vi "MIMIC Commands Rev 6.vi"(6 "MIMIC HOST COMMAND":T2(ring)=enum."Read Serial Number", 8 "Input String Data Array":string[](array[string])=["1"], 9 "HWHSflag":bool, 10 "wait (ms)":u32=500, 11 "VISA resource name":refnum<visa-resource-name>="COM5") -> (0 "error out":errorcluster={"status"=FALSE, "code"=1073676294, "source"="VISA Read in MIMIC RecvCommand.vi->MIMIC Commands Rev 2.vi"}, 1 "Receive_buffer":u8[](array[numeric]) format="%x", 2 "Receive_Unpacked_Data":T1)   [LabVIEW 2014]
panel:
  out "local":i32
  out "GUID":string
  out "Array":u8[](array[numeric]) format="%x"
  out "TimeToDecode":u16
  out "VISA resource name OUT":refnum<visa-resource-name>="COM5"
  out "hex integer string":string[](array[string])=["4", "D0", "0", "0", "FF", "2C"]
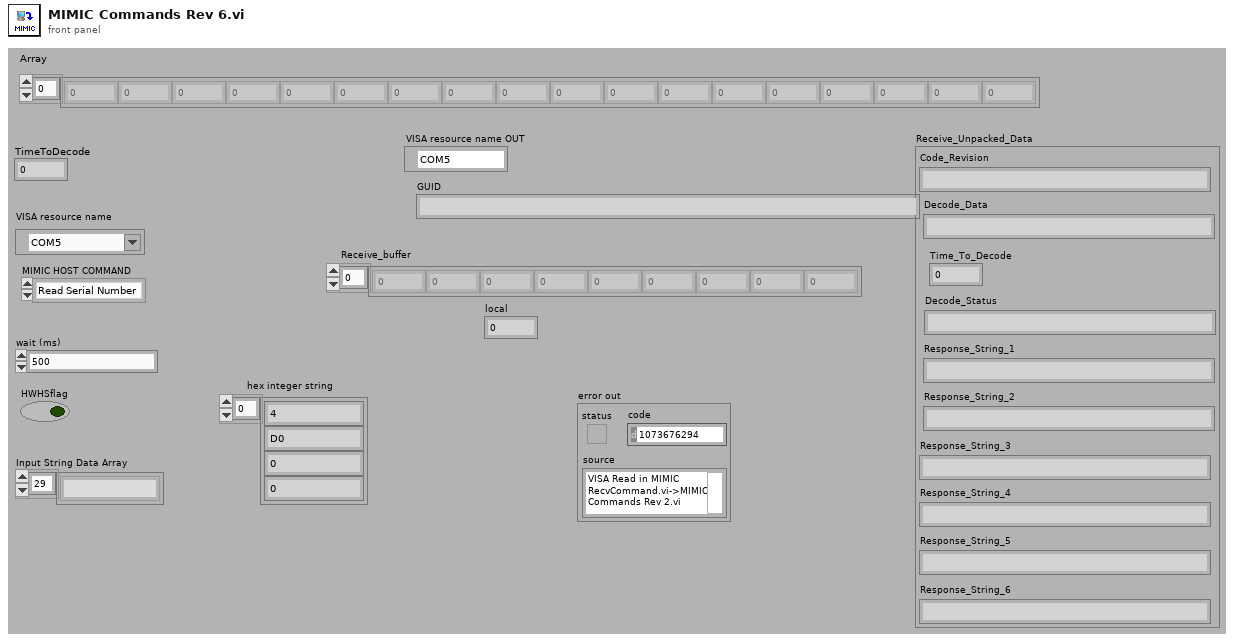
[diagram p1: front panel]
types:
  T1 = cluster{"Code_Revision":string, "Decode_Data":string, "Decode_Status":string, "Response_String_1":string, "Response_String_2":string, "Response_String_3":string, "Response_String_4":string, "Response_String_5":string, "Response_String_6":string, "Time_To_Decode":u16}
  T2 = enum16{"Enter FAT", "Beeper Control", "LED Off", "LED On", "Image Mode", "Start Session", "Stop Session", "Change Buadrate", "Auto Exposure", "Set Manual Exposure", "Read BT Address", "Store BT Address", "Pairing Command", "Query Paired Address", "Pairing Status", "Un-Pairing", "Set Illumination", "Trigger", "Set Defaults", "Imager Time To Decode Test", "Battery Off", "Battery Charge Control", "Read Battery Voltage", "Read Battery Temperature", "Software Version", "StoreFeatureSet", "ReadFeatureSet", "Store Model Number", "Read Model Number", "Store Manufacturing Date", "Read Manufacturing Date", "Store Service Date", "Read Service Date", "Store Serial Number", "Read Serial Number", "Exit FAT", "Read GUID", "Cable Auto ID", "Store RSM 627", "Read RSM 627", "Hall Effect switch", "Store GUID ", "ParamSend", "General", "General-Response", "RSM Init", "RSM EnterFAT", "RSM - SE4500 - Peek PRISM Register GENERIC command", "RSM - SE4500 - Poke PRISM Register GENERIC command", "RSM - SE4500 - GENERIC command", "RSM - SE4500 - GetPDM Calibration", "RSM - SE4500 - SetPDM Calibration", "Get Object Sensor Value", "Store Object Sensor Calibration Value", "Read Object Sensor Calibration Value", "RSM - SE4500 - GetPDM-Z Calibration", "RSM - SE4500 - SetPDM-Z Calibration", "Store FIPSKEY", "Read FIPSKEY"}
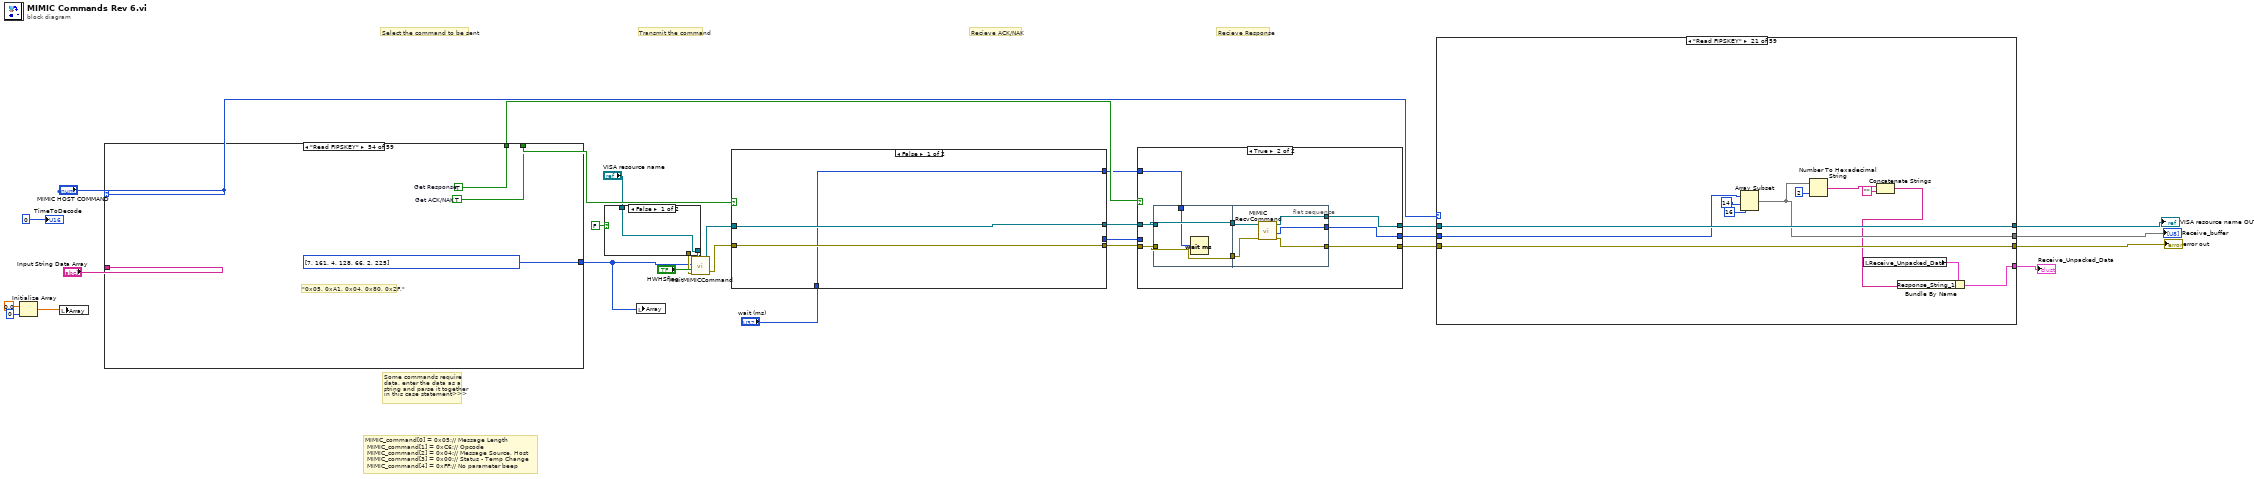
[diagram p0: block diagram]
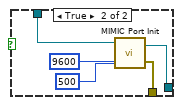
[diagram p2: hidden frame]
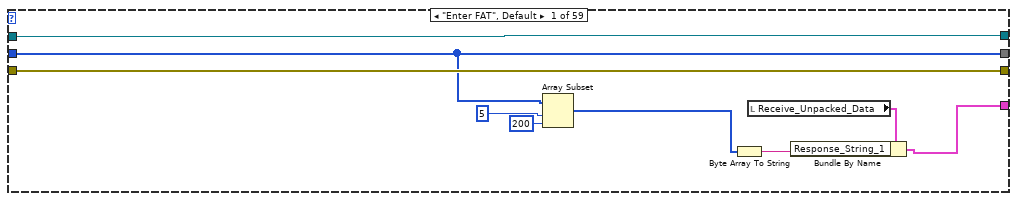
[diagram p3: hidden frame]
diagram:
  # "MIMIC_command[0] = 0x05;// Message Length \n\tMIMIC_command[1] = 0xC6;// Opcode  \n\tMIMIC_command[2] = 0x04;// Message Source, Host \n\tMIMIC_command[3] = 0x00;// Status - Temp Change            \n\tMIMIC_command[4] = 0xFF;// No parameter beep"
  # "Transmit the command"
  # "Recieve Response"
  # "Recieve ACK/NAK"
  # "Select the command to be sent"
  # "Some commands require\ndata, enter the data as a\nstring and parse it together\nin this case statement>>>"
  n1 = Initialize Array(0.0 ("element"), 0 ("dimension size")) -> (w5:dbl[])
  n2 = local write "Array"(w5) -> ()
  n3 = case shown="\"Read FIPSKEY\"" "MIMIC HOST COMMAND" {
    tunnel: "Input String Data Array" -> [w37 w39 w62 _ _ _ _ _ w86 w113 w139 w179 w219 w256 _ _ _ w274 w290 w300 w315 w328 w346 w362 _ _ _ _ _ w386 _ _ _ w406 _ _ _ _ w431 _ w443 _ w453 _ _ _ w479 _ w491 _ _ _ _ _ _ _ _ _ _]
    tunnel: [w31 w45 w66 u8[] [5, 161, 4, 128, 16, 0, 0, 0, 0, 0, 0, 0, 0, 0] u8[] [14, 128, 4, 0, 0, 10, 112, 0, 1, 20, 112, 12, 0, 132] u8[] [14, 128, 4, 0, 0, 10, 112, 0, 1, 20, 112, 31, 0, 113] u8[] [12, 128, 4, 0, 0, 6, 32, 0, 0, 240, 0, 0, 0, 0] u8[] [13, 128, 4, 0, 0, 9, 112, 0, 1, 2, 120, 1, 135, 0] w85 w119 w140 w176 w217 w257 u8[] [4, 228, 4, 0, 0, 0, 0, 0, 0, 0, 0, 0, 0, 0] u8[] [4, 228, 4, 0, 0, 0, 0, 0, 0, 0, 0, 0, 0, 0] u8[] [7, 215, 4, 0, 4, 11, 0, 255, 15, 0, 0, 0, 0, 0] w275 w284 w298 w313 w332 w349 w361 u8[] [16, 161, 4, 128, 16, 0, 0, 0, 0, 0, 0, 0, 0, 0] u8[] [5, 161, 4, 128, 16, 0, 0, 0, 0, 0, 0, 0, 0, 0] u8[] [4, 200, 4, 128, 0, 0, 0, 0, 0, 0, 0, 0, 0, 0] u8[] [5, 161, 4, 128, 25, 0, 0, 0, 0, 0, 0, 0, 0, 0] u8[] [7, 161, 4, 128, 66, 2, 29, 0, 0, 0, 0, 0, 0, 0] w385 u8[] [6, 161, 4, 128, 45, 2, 0, 0, 0, 0, 0, 0, 0, 0] u8[] [7, 161, 4, 128, 48, 19, 136, 0, 0, 0, 0, 0, 0, 0] u8[] [5, 161, 4, 128, 60, 0, 0, 0, 0, 0, 0, 0, 0, 0] w405 u8[] [7, 161, 4, 128, 66, 117, 48, 0, 0, 0, 0, 0, 0, 0] u8[] [7, 161, 4, 128, 66, 117, 49, 0, 0, 0, 0, 0, 0, 0] u8[] [7, 161, 4, 128, 66, 78, 41, 0, 0, 0, 0, 0, 0, 0] u8[] [6, 161, 4, 128, 96, 8] w424 u8[] [7, 161, 4, 128, 66, 3, 36] w445 u8[] [7, 161, 4, 128, 66, 2, 194, 0, 0, 0, 0, 0, 0, 0] w458 u8[] [7, 161, 4, 128, 66, 2, 21, 0, 0, 0, 0, 0, 0, 0] w472 u8[] [7, 161, 4, 128, 66, 2, 23, 0, 0, 0, 0, 0, 0, 0] w484 u8[] [7, 161, 4, 128, 66, 2, 24, 0, 0, 0, 0, 0, 0, 0] w496 u8[] [7, 161, 4, 128, 66, 2, 22, 0, 0, 0, 0, 0, 0, 0] u8[] [5, 161, 4, 128, 54, 254, 160, 0, 0, 0, 0, 0, 0, 0] u8[] [5, 161, 4, 128, 84, 0, 0, 0, 0, 0, 0, 0, 0, 0] u8[] [5, 161, 4, 128, 47] u8[] [7, 161, 4, 128, 66, 2, 225] w514 u8[] [5, 161, 4, 128, 110] u8[] [10, 161, 4, 128, 69, 2, 115, 66, 7, 2] u8[] [6, 161, 4, 128, 45, 1, 0, 0, 0, 0, 0, 0, 0, 0] u8[] [7, 161, 4, 128, 66, 2, 115]] -> w6
    tunnel: [w30 w57 w64 w71 w75 w78 w81 w84 w108 w135 w172 w192 w232 w258 w266 w269 w271 w276 w291 w301 w316 w333 w350 w368 w371 w373 w376 w380 w384 w388 w395 w399 w402 w403 w414 w417 w419 w422 w437 w440 w448 w451 w457 w462 w471 w476 w483 w487 w494 w499 w503 w507 w508 w511 w519 w521 w524 w527 w531] -> w25
    tunnel: [w29 w56 w65 w70 w74 w77 w80 w83 w107 w134 w171 w191 w231 w259 w267 w270 w272 w277 w292 w302 w317 w334 w351 w369 w372 w374 w377 w379 w383 w387 w396 w398 w401 w404 w413 w416 w418 w421 w436 w439 w447 w450 w456 w463 w470 w475 w482 w488 w495 w500 w502 w506 w509 w512 w520 w522 w525 w528 w530] -> w27
    frame "LED On" {
      w30 = FALSE  # Get Response
      w29 = TRUE  # Get ACK/NAK
      # "LED data Byte"
      n4 = Index Array(array=w37, index=0) -> (element=w36:string)
      n5 = Decimal String To Number(string=w36) -> (number=w35:i32)  [unwired: 2 in, 1 out]
      n6 = Replace Array Subset(array=u8[] [5, 231, 4, 128, 1, 0, 0, 0, 0, 0, 0, 0, 0, 0], new element=w35, index=4) -> (w31:u8[])
    }
    frame "ParamSend" {
      w57 = FALSE  # Get Response
      w56 = TRUE  # Get ACK/NAK
      n7 = Array Size(array=w39) -> (size(s)=w38:i32)
      n8 = Index Array(array=w39, index=0) -> (element=w61:string)
      n9 = Add(x=w38, y=5) -> (x+y=w43:i32)
      n10 = Hexadecimal String To Number(string=w61) -> (number=w42:u32)  [unwired: 2 in, 1 out]
      n11 = Replace Array Subset(array=u8[] [5, 198, 4, 128, 255, 0, 0, 0, 0, 0, 0, 0, 0, 0], new element=w43, index=0) -> (w54:u8[])
      n12 = Replace Array Subset(array=w54, new element=w42, index=5) -> (w50:u8[])
      n13 = Index Array(array=w39, index=2) -> (element=w49:string)
      n14 = Index Array(array=w39, index=1) -> (element=w53:string)
      n15 = Hexadecimal String To Number(string=w49) -> (number=w40:u32)  [unwired: 2 in, 1 out]
      n16 = Hexadecimal String To Number(string=w53) -> (number=w41:u32)  [unwired: 2 in, 1 out]
      n17 = Replace Array Subset(array=w50, new element=w41, index=6) -> (w46:u8[])
      n18 = Replace Array Subset(array=w46, new element=w40, index=7) -> (w45:u8[])
    }
    frame "Beeper Control" {
      w64 = FALSE  # Get Response
      w65 = TRUE  # Get ACK/NAK
      # "Beeper data Byte"
      n19 = Decimal String To Number(string=w62, offset=0) -> (number=w69:i32[])  [unwired: 1 in, 1 out]
      n20 = Replace Array Subset(array=u8[] [5, 230, 4, 128, 0, 0, 0, 0, 0, 0, 0, 0, 0, 0], new element=w69, index=4) -> (w66:u8[])
    }
    frame "Enter FAT" {
      w71 = TRUE  # Get Response
      w70 = TRUE  # Get ACK/NAK
      # "Enter FAT command:\n0x05:0xA1:0x40:0x80:0x10"
    }
    frame "RSM - SE4500 - GetPDM Calibration" {
      w75 = TRUE  # Get Response
      w74 = FALSE  # Get ACK/NAK
      # "RSM GetDPMCalibration Command"
    }
    frame "RSM - SE4500 - GetPDM-Z Calibration" {
      w78 = TRUE  # Get Response
      w77 = FALSE  # Get ACK/NAK
      # "RSM GetDPMCalibration Command"
    }
    frame "RSM Init" {
      w81 = TRUE  # Get Response
      w80 = FALSE  # Get ACK/NAK
      # "Init RSM command:\n0x0C:0x80:0x04:0x00:0x00:0x06:0x20:0x00:0x00:0xF0"
    }
    frame "RSM EnterFAT" {
      w84 = TRUE  # Get Response
      w83 = FALSE  # Get ACK/NAK
      # "RSM / SE4500 - Enter FAT command:\n0x0D:0x80:0x04:0x00:0x00:0x09:0x70:0x00:0x01:0x02:0x78:0x01:0x87:"
    }
    frame "RSM - SE4500 - Peek PRISM Register GENERIC command" {
      w108 = TRUE  # Get Response
      w107 = FALSE  # Get ACK/NAK
      # "Register Word - HEX String"
      # "RSM / SE4500 - Peek PRISM Register GENERIC command:\n0x0E:0x80:0x04:0x00:0x00:0x0B:0x70:0x00:0x01:0x02:0xC3:0xXX:0xXX:0xXX:0xCS"
      n21 = Index Array(array=w86, index=0) -> (element=w90:string)
      n22 = Hexadecimal String To Number(string=w90, default (0uL)=i16 0 ("default (0 I32)")) -> (number=w88:i16)  [unwired: 1 in, 1 out]
      n23 = Split Number(x=w88) -> (hi(x)=w94:u8, lo(x)=w92:u8)
      n24 = Replace Array Subset(array=u8[] [15, 128, 4, 0, 0, 11, 112, 0, 1, 3, 195, 0, 0, 0, 0], new element=w94, index=11) -> (w91:u8[])
      n25 = Replace Array Subset(array=w91, new element=w92, index=12) -> (w87:u8[])
      n26 = Array Subset(array=w87, index=10, length=3) -> (w97:u8[])
      n27 = for {
        N: 3 -> [_]
        tunnel: w97 -> [w111] mode=indexing
        shift-right: [w109] -> w103
        shift-left: u16 0 -> [w110]
        n28 = Add(x=w110, y=w111) -> (x+y=w109:u16)
      }
      n29 = Not(x=w103) -> (.not. x?=w102:u16)
      n30 = Increment(x=w102) -> (x+1=w101:u16)
      n31 = Replace Array Subset(array=w87, new element=w101, index=13) -> (w85:u8[])
    }
    frame "RSM - SE4500 - GENERIC command" {
      w114 = 1 ("index")
      w118 = 0 ("index")
      w135 = TRUE  # Get Response
      w134 = FALSE  # Get ACK/NAK
      # "Register Word - HEX String"
      # "RSM / SE4500 - Peek PRISM Register GENERIC command:\n0x0E:0x80:0x04:0x00:0x00:0x0B:0x70:0x00:0x01:0x02:0xXX:0xXX:0xXX:0xCS"
      n32 = Index Array(array=w113, index=w118) -> (element=w121:string)
      n33 = Index Array(array=w113, index=w114) -> (element=w115:string)
      n34 = Hexadecimal String To Number(string=w121, default (0uL)=w118) -> (number=w116:i32)  [unwired: 1 in, 1 out]
      n35 = Hexadecimal String To Number(string=w115, default (0uL)=w114) -> (number=w112:i32)  [unwired: 1 in, 1 out]
      n36 = Replace Array Subset(array=u8[] [13, 128, 4, 0, 0, 9, 112, 0, 1, 2, 255, 0, 0], new element=w116, index=10) -> (w122:u8[])
      n37 = Replace Array Subset(array=w122, new element=w112, index=11) -> (w120:u8[])
      n38 = Array Subset(array=w120, index=10, length=2) -> (w125:u8[])
      n39 = for {
        N: 2 -> [_]
        tunnel: w125 -> [w138] mode=indexing
        shift-right: [w136] -> w131
        shift-left: u16 0 -> [w137]
        n40 = Add(x=w137, y=w138) -> (x+y=w136:u16)
      }
      n41 = Not(x=w131) -> (.not. x?=w130:u16)
      n42 = Increment(x=w130) -> (x+1=w129:u16)
      n43 = Replace Array Subset(array=w120, new element=w129, index=12) -> (w119:u8[])
    }
    frame "RSM - SE4500 - Poke PRISM Register GENERIC command" {
      w172 = TRUE  # Get Response
      w171 = FALSE  # Get ACK/NAK
      # "Register Word - HEX String"
      # "Register Word - HEX String"
      # "Value Byte - Decimal String"
      # "RSM / SE4500 - Poke PRISM Register GENERIC command:\n0x0E:0x80:0x04:0x00:0x00:0x0B:0x70:0x00:0x01:0x02:0xC0:0xXX:0xXX:0xXX:0xCS"
      n44 = Index Array(array=w139, index=0) -> (element=w154:string)
      n45 = Index Array(array=w139, index=1) -> (element=w145:string)
      n46 = Hexadecimal String To Number(string=w154, default (0uL)=i16 0 ("default (0 I32)")) -> (number=w152:i16)  [unwired: 1 in, 1 out]
      n47 = Split Number(x=w152) -> (hi(x)=w158:u8, lo(x)=w156:u8)
      n48 = Hexadecimal String To Number(string=w145, default (0uL)=i16 0 ("default (0 I32)")) -> (number=w151:i16)  [unwired: 1 in, 1 out]
      n49 = Replace Array Subset(array=u8[] [16, 128, 4, 0, 0, 12, 112, 0, 1, 2, 151, 0, 0, 0, 0, 0], new element=w158, index=12) -> (w155:u8[])
      n50 = Split Number(x=w151) -> (hi(x)=w148:u8, lo(x)=w150:u8)
      n51 = Replace Array Subset(array=w155, new element=w156, index=11) -> (w143:u8[])
      n52 = Replace Array Subset(array=w143, new element=w148, index=14) -> (w142:u8[])
      n53 = Replace Array Subset(array=w142, new element=w150, index=13) -> (w141:u8[])
      n54 = Array Subset(array=w141, index=10, length=5) -> (w161:u8[])
      n55 = for {
        N: 5 -> [_]
        tunnel: w161 -> [w175] mode=indexing
        shift-right: [w173] -> w167
        shift-left: u16 0 -> [w174]
        n56 = Add(x=w174, y=w175) -> (x+y=w173:u16)
      }
      n57 = Not(x=w167) -> (.not. x?=w166:u16)
      n58 = Increment(x=w166) -> (x+1=w165:u16)
      n59 = Replace Array Subset(array=w141, new element=w165, index=15) -> (w140:u8[])
    }
    frame "RSM - SE4500 - SetPDM Calibration" {
      w192 = TRUE  # Get Response
      w191 = FALSE  # Get ACK/NAK
      # "RSM / SE4500 - SetDPMCalibration command:"
      n60 = for {
        N: 8 -> [_]
        shift-right: [w202] -> w178
        shift-left: u8[] [30, 128, 4, 0, 0, 26, 112, 0, 1, 2, 148, 12, 0, 0, 0, 0, 0, 0, 0, 0, 0, 0, 0, 0, 0, 0, 0, 0, 0, 0, 0] -> [w209]
        tunnel: w179 -> [w208]
        i -> [w204]
        # "high byte"
        # "low byte"
        n61 = Index Array(array=w208, index=w204) -> (element=w197:string)
        n62 = Decimal String To Number(string=w197, default (0L)=0 ("default (0 I32)")) -> (number=w194:i32)  [unwired: 1 in, 1 out]
        n63 = Number To Hexadecimal String(1:i16 4 ("width (-)"), 2:w194) -> (0:w195:string)
        n64 = local read "local"() -> (w200:i32)
        n65 = Hexadecimal String To Number(string=w195, default (0uL)=i16 0 ("default (0 I32)")) -> (number=w210:i16)  [unwired: 1 in, 1 out]
        n66 = Add(x=1 ("y"), y=w200) -> (x+y=w198:i32)
        n67 = Add(x=w204, y=w198) -> (x+y=w201:i32)
        n68 = Add(x=1 ("index"), y=w201) -> (x+y=w206:i32)
        n69 = Split Number(x=w210) -> (hi(x)=w212:u8, lo(x)=w211:u8)
        n70 = Replace Array Subset(array=w209, new element=w212, index=w206) -> (w203:u8[])
        n71 = local write "local"(w198) -> ()
        n72 = Replace Array Subset(array=w203, new element=w211, index=w201) -> (w202:u8[])
      }
      n73 = Array Subset(array=w178, index=10, length=19) -> (w182:u8[])
      n74 = for {
        N: 19 -> [_]
        tunnel: w182 -> [w215] mode=indexing
        shift-right: [w213] -> w188
        shift-left: u16 0 -> [w214]
        n75 = Add(x=w214, y=w215) -> (x+y=w213:u16)
      }
      n76 = Not(x=w188) -> (.not. x?=w187:u16)
      n77 = Increment(x=w187) -> (x+1=w186:u16)
      n78 = Replace Array Subset(array=w178, new element=w186, index=29) -> (w176:u8[])
      "local" <- 12 ("x+y")
    }
    frame "RSM - SE4500 - SetPDM-Z Calibration" {
      w232 = TRUE  # Get Response
      w231 = FALSE  # Get ACK/NAK
      # "RSM / SE4500 - SetDPMCalibration command:"
      n79 = local write "local"(12 ("x+y")) -> ()
      n80 = for {
        N: 8 -> [_]
        shift-right: [w242] -> w218
        shift-left: u8[] [30, 128, 4, 0, 0, 26, 112, 0, 1, 2, 148, 31, 0, 0, 0, 0, 0, 0, 0, 0, 0, 0, 0, 0, 0, 0, 0, 0, 0, 0, 0] -> [w249]
        tunnel: w219 -> [w248]
        i -> [w244]
        # "high byte"
        # "low byte"
        n81 = Index Array(array=w248, index=w244) -> (element=w237:string)
        n82 = Decimal String To Number(string=w237, default (0L)=0 ("default (0 I32)")) -> (number=w234:i32)  [unwired: 1 in, 1 out]
        n83 = Number To Hexadecimal String(1:i16 4 ("width (-)"), 2:w234) -> (0:w235:string)
        n84 = local read "local"() -> (w240:i32)
        n85 = Hexadecimal String To Number(string=w235, default (0uL)=i16 0 ("default (0 I32)")) -> (number=w250:i16)  [unwired: 1 in, 1 out]
        n86 = Add(x=1 ("y"), y=w240) -> (x+y=w238:i32)
        n87 = Add(x=w244, y=w238) -> (x+y=w241:i32)
        n88 = Add(x=1 ("index"), y=w241) -> (x+y=w246:i32)
        n89 = Split Number(x=w250) -> (hi(x)=w252:u8, lo(x)=w251:u8)
        n90 = Replace Array Subset(array=w249, new element=w252, index=w246) -> (w243:u8[])
        n91 = local write "local"(w238) -> ()
        n92 = Replace Array Subset(array=w243, new element=w251, index=w241) -> (w242:u8[])
      }
      n93 = Array Subset(array=w218, index=10, length=19) -> (w222:u8[])
      n94 = for {
        N: 19 -> [_]
        tunnel: w222 -> [w255] mode=indexing
        shift-right: [w253] -> w228
        shift-left: u16 0 -> [w254]
        n95 = Add(x=w254, y=w255) -> (x+y=w253:u16)
      }
      n96 = Not(x=w228) -> (.not. x?=w227:u16)
      n97 = Increment(x=w227) -> (x+1=w226:u16)
      n98 = Replace Array Subset(array=w218, new element=w226, index=29) -> (w217:u8[])
    }
    frame "Image Mode" {
      w258 = FALSE  # Get Response
      w259 = TRUE  # Get ACK/NAK
      # "Image Mode Byte:\n00: Decode\n01: SnapShot\n02: Video\n03: Last Decode\n04: las No Decode"
      n99 = Index Array(array=w256, index=0) -> (element=w264:string)
      n100 = Decimal String To Number(string=w264) -> (number=w263:i32)  [unwired: 2 in, 1 out]
      n101 = Replace Array Subset(array=u8[] [5, 247, 4, 128, 0, 0, 0, 0, 0, 0, 0, 0, 0, 0], new element=w263, index=4) -> (w257:u8[])
    }
    frame "Start Session" {
      w266 = FALSE  # Get Response
      w267 = TRUE  # Get ACK/NAK
      # "Start Session"
    }
    frame "Stop Session" {
      w269 = FALSE  # Get Response
      w270 = TRUE  # Get ACK/NAK
      # "Start Session"
    }
    frame "Change Buadrate" {
      w271 = FALSE  # Get Response
      w272 = FALSE  # Get ACK/NAK
      # "Enter FAT command:\n06: 9600\n08: 38400\n0A: 57600\n0B:115200\n0C:230400"
    }
    frame "Auto Exposure" {
      w276 = FALSE  # Get Response
      w277 = TRUE  # Get ACK/NAK
      # "Auto Exposure:\n00:Disabled\n01: Enabled"
      n102 = Index Array(array=w274, index=0) -> (element=w282:string)
      n103 = Decimal String To Number(string=w282) -> (number=w281:i32)  [unwired: 2 in, 1 out]
      n104 = Replace Array Subset(array=u8[] [8, 198, 4, 0, 255, 240, 41, 0, 0, 0, 0, 0, 0, 0], new element=w281, index=7) -> (w275:u8[])
    }
    frame "Set Manual Exposure" {
      w291 = FALSE  # Get Response
      w292 = TRUE  # Get ACK/NAK
      # "Image Mode Byte:\n00: Decode\n01: SnapShot\n02: Video\n03: Last Decode\n04: las No Decode"
      n105 = Index Array(array=w290, index=0) -> (element=w296:string)
      n106 = Decimal String To Number(string=w296, default (0L)=u16 0 ("default (0 I32)")) -> (number=w289:u16)  [unwired: 1 in, 1 out]
      n107 = Split Number(x=w289) -> (hi(x)=w287:u8, lo(x)=w286:u8)
      n108 = Replace Array Subset(array=u8[] [10, 198, 4, 0, 255, 244, 241, 55, 0, 0, 0, 0, 0, 0], new element=w287, index=8) -> (w283:u8[])
      n109 = Replace Array Subset(array=w283, new element=w286, index=9) -> (w284:u8[])
    }
    frame "Store BT Address" {
      w301 = FALSE  # Get Response
      w302 = TRUE  # Get ACK/NAK
      # "Store BT command:\n0x16, 0xA1, 0x04, 0x80, 0x45, 0x02, 0x1D, 0x41, 0x07, 0x42, 0x00, 0x06, 0x00, 0x00, \n\t\t\t\t\t\t\t\t\t\t0x00, 0x00, 0x00, 0x00, 0x00, 0x00,0x00, 0x00, 0xFF, 0xFF};"
      n110 = for {
        N: 6 -> [_]
        tunnel: w300 -> [w311]
        tunnel: [w306] -> w298
        i -> [w308]
        n111 = Index Array(array=w311, index=w308) -> (element=w305:string)
        n112 = Add(x=14 ("index"), y=w308) -> (x+y=w309:i32)
        n113 = Hexadecimal String To Number(string=w305, offset=0) -> (number=w303:u32)  [unwired: 1 in, 1 out]
        n114 = local read "Array"() -> (w307:u8[])
        n115 = Replace Array Subset(array=w307, new element=w303, index=w309) -> (w306:u8[])
        n116 = local write "Array"(w306) -> ()
      }
      "Array" <- u8[] [22, 161, 4, 128, 69, 2, 29, 65, 7, 66, 0, 6, 0, 0, 0, 0, 0, 0, 0, 0, 255, 255, 255, 0, 0, 0, 0, 0, 0, 0, 0, 0, 0, 0, 0, 0, 0, 0, 0, 0, 0, 0, 0, 0, 0, 0, 0, 0, 0, 0, 0]
    }
    frame "Store FIPSKEY" {
      w316 = FALSE  # Get Response
      w317 = TRUE  # Get ACK/NAK
      # "Store BT command:\n0x20, 0xA1, 0x04, 0x80, 0x45, 0x02, 0xE1, 0x41, 0x07, 0x42, 0x00, 0x16, 0x00, 0x00,"
      n117 = for {
        N: 16 -> [_]
        tunnel: w315 -> [w326]
        tunnel: [w321] -> w313
        i -> [w323]
        n118 = Index Array(array=w326, index=w323) -> (element=w320:string)
        n119 = Add(x=14 ("index"), y=w323) -> (x+y=w324:i32)
        n120 = Hexadecimal String To Number(string=w320, offset=0) -> (number=w318:u32)  [unwired: 1 in, 1 out]
        n121 = local read "Array"() -> (w322:u8[])
        n122 = Replace Array Subset(array=w322, new element=w318, index=w324) -> (w321:u8[])
        n123 = local write "Array"(w321) -> ()
      }
      n124 = local write "Array"(u8[] [32, 161, 4, 128, 69, 2, 225, 65, 7, 66, 0, 22, 0, 0, 0, 0, 0, 0, 0, 0, 255, 255, 255, 0, 0, 0, 0, 0, 0, 0, 0, 0, 0, 0, 0, 0, 0, 0, 0, 0, 0, 0, 0, 0, 0, 0, 0, 0, 0, 0, 0]) -> ()
    }
    frame "General" {
      w330 = 0 ("offset")
      w333 = FALSE  # Get Response
      w334 = TRUE  # Get ACK/NAK
      # "Gneral FAT command:\n0x16, 0xA1, 0x04, 0x80, 0x45, 0x02, 0x1D, 0x41, 0x07, 0x42, 0x00, 0x06, 0x00, 0x00, \n\t\t\t\t\t\t\t\t\t\t0x00, 0x00, 0x00, 0x00, 0x00, 0x00,0x00, 0x00, 0xFF, 0xFF};"
      n125 = Index Array(array=w328, index=w330) -> (element=w329:string)
      n126 = Hexadecimal String To Number(string=w329, offset=w330) -> (number=w327:u32)  [unwired: 1 in, 1 out]
      n127 = for {
        N: w327 -> [_]
        tunnel: w328 -> [w343]
        tunnel: [w338] -> w332
        i -> [w340]
        n128 = Index Array(array=w343, index=w340) -> (element=w337:string)
        n129 = Add(x=0 ("index"), y=w340) -> (x+y=w341:i32)
        n130 = Hexadecimal String To Number(string=w337, offset=0) -> (number=w335:u32)  [unwired: 1 in, 1 out]
        n131 = local read "Array"() -> (w339:u8[])
        n132 = Replace Array Subset(array=w339, new element=w335, index=w341) -> (w338:u8[])
        n133 = local write "Array"(w338) -> ()
      }
      n134 = local write "Array"(u8[] [22, 0, 0, 0, 0, 0, 0, 0, 0, 0, 0, 0, 0, 0, 0, 0, 0, 0, 0, 0, 0, 0, 0, 0, 0, 0, 0, 0, 0, 0, 0, 0, 0, 0, 0, 0, 0, 0, 0, 0, 0, 0, 0, 0, 0, 0, 0, 0, 0, 0, 0]) -> ()
    }
    frame "General-Response" {
      w345 = 0 ("offset")
      w350 = TRUE  # Get Response
      w351 = TRUE  # Get ACK/NAK
      # "Gneral FAT command:\n0x16, 0xA1, 0x04, 0x80, 0x45, 0x02, 0x1D, 0x41, 0x07, 0x42, 0x00, 0x06, 0x00, 0x00, \n\t\t\t\t\t\t\t\t\t\t0x00, 0x00, 0x00, 0x00, 0x00, 0x00,0x00, 0x00, 0xFF, 0xFF};"
      n135 = Index Array(array=w346, index=w345) -> (element=w344:string)
      n136 = Hexadecimal String To Number(string=w344, offset=w345) -> (number=w347:u32)  [unwired: 1 in, 1 out]
      n137 = for {
        N: w347 -> [_]
        tunnel: w346 -> [w360]
        tunnel: [w355] -> w349
        i -> [w357]
        n138 = Index Array(array=w360, index=w357) -> (element=w354:string)
        n139 = Add(x=0 ("index"), y=w357) -> (x+y=w358:i32)
        n140 = Hexadecimal String To Number(string=w354, offset=0) -> (number=w352:u32)  [unwired: 1 in, 1 out]
        n141 = local read "Array"() -> (w356:u8[])
        n142 = Replace Array Subset(array=w356, new element=w352, index=w358) -> (w355:u8[])
        n143 = local write "Array"(w355) -> ()
      }
      n144 = local write "Array"(u8[] [22, 0, 0, 0, 0, 0, 0, 0, 0, 0, 0, 0, 0, 0, 0, 0, 0, 0, 0, 0, 0, 0, 0, 0, 0, 0, 0, 0, 0, 0, 0, 0, 0, 0, 0, 0, 0, 0, 0, 0, 0, 0, 0, 0, 0, 0, 0, 0, 0, 0, 0]) -> ()
    }
    frame "Pairing Command" {
      w368 = TRUE  # Get Response
      w369 = FALSE  # Get ACK/NAK
      # "Pairing  command:\n10 9E 04 80 00 00 02 03 06 08  01 0B 03 00 0F 0F FE 8E"
      n145 = Index Array(array=w362, index=0) -> (element=w366:string)
      n146 = String To Byte Array(string=w366) -> (unsigned byte array=w364:u8[])
      n147 = Replace Array Subset(array=u8[] [16, 158, 4, 128, 0, 0, 0, 0, 0, 8, 1, 11, 3, 0, 15, 15], new element=w364, index=4) -> (w361:u8[])
    }
    frame "Un-Pairing" {
      w371 = TRUE  # Get Response
      w372 = FALSE  # Get ACK/NAK
      # "Enter FAT command:\n0x05:0xA1:0x40:0x80:0x10"
    }
    frame "Set Illumination" {
      w373 = TRUE  # Get Response
      w374 = FALSE  # Get ACK/NAK
      # "Enter FAT command:\n0x05:0xA1:0x40:0x80:0x10"
    }
    frame "Set Defaults" {
      w376 = FALSE  # Get Response
      w377 = TRUE  # Get ACK/NAK
    }
    frame "Exit FAT" {
      w380 = TRUE  # Get Response
      w379 = TRUE  # Get ACK/NAK
    }
    frame "Read BT Address" {
      w384 = TRUE  # Get Response
      w383 = TRUE  # Get ACK/NAK
    }
    frame "LED Off" {
      w388 = FALSE  # Get Response
      w387 = TRUE  # Get ACK/NAK
      # "LED data Byte"
      n148 = Index Array(array=w386, index=0) -> (element=w393:string)
      n149 = Decimal String To Number(string=w393) -> (number=w392:i32)  [unwired: 2 in, 1 out]
      n150 = Replace Array Subset(array=u8[] [5, 232, 4, 128, 1, 0, 0, 0, 0, 0, 0, 0, 0, 0], new element=w392, index=4) -> (w385:u8[])
    }
    frame "Trigger" {
      w395 = TRUE  # Get Response
      w396 = TRUE  # Get ACK/NAK
    }
    frame "Imager Time To Decode Test" {
      w399 = TRUE  # Get Response
      w398 = TRUE  # Get ACK/NAK
      # "Start Session"
    }
    frame "Battery Off" {
      w402 = FALSE  # Get Response
      w401 = TRUE  # Get ACK/NAK
      # "Enter FAT command:\n0x05:0xA1:0x40:0x80:0x10"
    }
    frame "Battery Charge Control" {
      w403 = FALSE  # Get Response
      w404 = TRUE  # Get ACK/NAK
      # "Battery Charge\n0x06, 0xA1, 0x04, 0x80, 0x3D\n0x00: Disable charging of battery\n0x01: Enable charging of battery\n0x02: Enable Slow charge (Hammer)"
      n151 = Index Array(array=w406, index=0) -> (element=w411:string)
      n152 = Decimal String To Number(string=w411) -> (number=w410:i32)  [unwired: 2 in, 1 out]
      n153 = Replace Array Subset(array=u8[] [6, 161, 4, 128, 61, 0, 0, 0, 0, 0, 0, 0, 0, 0], new element=w410, index=5) -> (w405:u8[])
    }
    frame "Read Battery Voltage" {
      w414 = TRUE  # Get Response
      w413 = FALSE  # Get ACK/NAK
      # "Read Battery Voltage command:\n0x07:0xA1:0x04:0x80:0x42:0x75:0x30"
    }
    frame "Read Battery Temperature" {
      w417 = TRUE  # Get Response
      w416 = FALSE  # Get ACK/NAK
      # "Read Battery Temperature command:\n0x07:0xA1:0x04:0x80:0x42:0x75:0x31"
    }
    frame "Software Version" {
      w419 = TRUE  # Get Response
      w418 = TRUE  # Get ACK/NAK
      # "Software Version command:\n\"0x07, 0xA1, 0x04, 0x80, 0x42, 0x4E, 0x29,\""
    }
    frame "Get Object Sensor Value" {
      w422 = TRUE  # Get Response
      w421 = TRUE  # Get ACK/NAK
      # "Get Object Sensor command:\n\"0x06,0xA1,0x04,0x80,0x60,0x08,\""
    }
    frame "Store Object Sensor Calibration Value" {
      w437 = FALSE  # Get Response
      w436 = TRUE  # Get ACK/NAK
      # "Store Object Sensor Calibration command:\n\"0x0B,0xA1,0x04,0x80,0x45,0x03,0x24,0x57,0x07,CAL H,CAL L"
      n154 = Index Array(array=w431, index=1) -> (element=w426:string)
      n155 = Index Array(array=w431, index=0) -> (element=w434:string)
      n156 = Hexadecimal String To Number(string=w434) -> (number=w427:u32)  [unwired: 2 in, 1 out]
      n157 = Hexadecimal String To Number(string=w426) -> (number=w425:u32)  [unwired: 2 in, 1 out]
      n158 = Replace Array Subset(array=u8[] [11, 161, 4, 128, 69, 3, 36, 87, 7, 0, 0], new element=w427, index=9) -> (w429:u8[])
      n159 = Replace Array Subset(array=w429, new element=w425, index=10) -> (w424:u8[])
    }
    frame "Read Object Sensor Calibration Value" {
      w440 = TRUE  # Get Response
      w439 = TRUE  # Get ACK/NAK
      # "Read Object Sensor Calibration command:\n\"0x07,0xA1,0x04,0x80,0x42,0x03,0x24,\""
    }
    frame "StoreFeatureSet" {
      w448 = FALSE  # Get Response
      w447 = TRUE  # Get ACK/NAK
      # "Store Feature Set command:\n\"0x0A, 0xA1, 0x04, 0x80, 0x45, 0x02, 0xC2, 0x42, 0x07,\n0xFF,//Feature Set Value \n0x00, 0x00}; //checksum\""
      n160 = Hexadecimal String To Number(string=w443, offset=0) -> (number=w441:u32[])  [unwired: 1 in, 1 out]
      n161 = Replace Array Subset(array=u8[] [10, 161, 4, 128, 69, 2, 194, 66, 7, 0, 0, 0, 0, 0], new element=w441, index=9) -> (w445:u8[])
    }
    frame "ReadFeatureSet" {
      w451 = TRUE  # Get Response
      w450 = TRUE  # Get ACK/NAK
      # "0x07, 0xA1, 0x04, 0x80, 0x42, 0x02, 0xC2, 0x00, 0x00};"
      # "Read Feature Set command:\n0x07, 0xA1, 0x04, 0x80, 0x42, 0x02, 0xC2,"
    }
    frame "Store Model Number" {
      w457 = FALSE  # Get Response
      w456 = TRUE  # Get ACK/NAK
      # "StoreModel Number command:\n0x20, 0xA1, 0x04, 0x80, 0x45, 0x02, 0x15, 0x53, 0x07, 0x00, 0x12, 0x00, 0x00,\n\t\t\t\t\t\t\t\t\t\t0x00, 0x00, 0x00, 0x00, 0x00, 0x00, 0x00, 0x00, 0x00,\n\t\t\t\t\t\t\t\t\t\t0x00, 0x00, 0x00, 0x00, 0x00, 0x00, 0x00, 0x00, 0x00,\n\t\t\t\t\t\t\t\t\t\t0x00"
      n162 = Index Array(array=w453, index=0) -> (element=w454:string)
      n163 = String To Byte Array(string=w454) -> (unsigned byte array=w455:u8[])
      n164 = Replace Array Subset(array=u8[] [32, 161, 4, 128, 69, 2, 21, 83, 7, 0, 18, 0, 0, 0, 0, 0, 0, 0, 0, 0, 0, 0, 0, 0, 0, 0, 0, 0, 0, 0, 0, 0, 0], new element=w455, index=13) -> (w458:u8[])
    }
    frame "Read Model Number" {
      w462 = TRUE  # Get Response
      w463 = TRUE  # Get ACK/NAK
      # "ReadModel Number command:\n0x07, 0xA1, 0x04, 0x80, 0x42, 0x02, 0x15,"
    }
    frame "Store Manufacturing Date" {
      w471 = FALSE  # Get Response
      w470 = TRUE  # Get ACK/NAK
      # "Store Manufacturing Date command:\n0x15, 0xA1, 0x04, 0x80, 0x45, 0x02, 0x17, 0x53, 0x07, 0x00, 0x07, 0x00, 0x00,\n\t\t\t\t\t\t\t\t\t\t0x00, 0x00, 0x00, 0x00, 0x00, 0x00, 0x00,\n\t\t\t\t\t\t\t\t\t\t0x00"
      n165 = Get Date/Time In Seconds() -> (seconds since 1Jan1904=w469:timestamp)
      n166 = Format Date/Time String(time format string (%c)="%d%b%y", seconds (now)=w469, UTC format=FALSE) -> (date/time string=w465:string)
      n167 = To Upper Case(1:w465) -> (0:w464:string)
      n168 = String To Byte Array(string=w464) -> (unsigned byte array=w466:u8[])
      n169 = Replace Array Subset(array=u8[] [21, 161, 4, 128, 69, 2, 23, 83, 7, 0, 7, 0, 0, 0, 0, 0, 0, 0, 0, 0, 0, 0], new element=w466, index=13) -> (w472:u8[])
    }
    frame "Read Manufacturing Date" {
      w476 = TRUE  # Get Response
      w475 = TRUE  # Get ACK/NAK
      # "Read Feature Set command:\n0x07, 0xA1, 0x04, 0x80, 0x42, 0x02, 0x17,"
    }
    frame "Store Service Date" {
      w483 = FALSE  # Get Response
      w482 = TRUE  # Get ACK/NAK
      # "StoreService Date command:\n0x15, 0xA1, 0x04, 0x80, 0x45, 0x02, 0x18, 0x53, 0x07, 0x00, 0x07, 0x00, 0x00,\n\t\t\t\t\t\t\t\t\t\t0x00, 0x00, 0x00, 0x00, 0x00, 0x00, 0x00,\n\t\t\t\t\t\t\t\t\t\t0x00"
      n170 = Index Array(array=w479, index=0) -> (element=w481:string)
      n171 = String To Byte Array(string=w481) -> (unsigned byte array=w478:u8[])
      n172 = Replace Array Subset(array=u8[] [21, 161, 4, 128, 69, 2, 24, 83, 7, 0, 7, 0, 0, 0, 0, 0, 0, 0, 0, 0, 0, 0], new element=w478, index=13) -> (w484:u8[])
    }
    frame "Read Service Date" {
      w487 = TRUE  # Get Response
      w488 = TRUE  # Get ACK/NAK
      # "Read Service Date command:\n0x07, 0xA1, 0x04, 0x80, 0x42, 0x02, 0x18,"
    }
    frame "Store Serial Number" {
      w494 = FALSE  # Get Response
      w495 = TRUE  # Get ACK/NAK
      # "Store Serial Number command:\n0x1E, 0xA1, 0x04, 0x80, 0x45, 0x02, 0x16, 0x53, 0x07, 0x00, 0x10, 0x00, 0x00,\n\t\t\t\t\t\t\t\t\t\t0x00, 0x00, 0x00, 0x00, 0x00, 0x00, 0x00, 0x00,\n\t\t\t\t\t\t\t\t\t\t0x00, 0x00, 0x00, 0x00, 0x00, 0x00, 0x00, 0x00,\n\t\t\t\t\t\t\t\t\t\t0x00"
      n173 = Index Array(array=w491, index=0) -> (element=w493:string)
      n174 = String To Byte Array(string=w493) -> (unsigned byte array=w490:u8[])
      n175 = Replace Array Subset(array=u8[] [30, 161, 4, 128, 69, 2, 22, 83, 7, 0, 16, 0, 0, 0, 0, 0, 0, 0, 0, 0, 0, 0, 0, 0, 0, 0, 0, 0, 0, 0, 0, 0, 0], new element=w490, index=13) -> (w496:u8[])
    }
    frame "Read Serial Number" {
      w499 = TRUE  # Get Response
      w500 = TRUE  # Get ACK/NAK
      # "Read Serial Number command:\n0x07, 0xA1, 0x04, 0x80, 0x42, 0x02, 0x16,"
    }
    frame "Pairing Status" {
      w503 = TRUE  # Get Response
      w502 = FALSE  # Get ACK/NAK
      # "Read Serial Number command:\n0x05, 0xA1, 0x04, 0x80, 0x36, 0xFE, 0xA0,"
    }
    frame "Query Paired Address" {
      w507 = TRUE  # Get Response
      w506 = FALSE  # Get ACK/NAK
      # "Read Serial Number command:\n0x05, 0xA1, 0x04, 0x80, 0x54,"
    }
    frame "Read GUID" {
      w508 = TRUE  # Get Response
      w509 = TRUE  # Get ACK/NAK
      # "\"0x05, 0xA1, 0x04, 0x80, 0x2F,\""
    }
    frame "Read FIPSKEY" {
      w511 = TRUE  # Get Response
      w512 = TRUE  # Get ACK/NAK
      # "\"0x05, 0xA1, 0x04, 0x80, 0x2F,\""
    }
    frame "Store GUID " {
      w519 = TRUE  # Get Response
      w520 = FALSE  # Get ACK/NAK
      # "32 bytes 0-9, A-F (0x30 - 0x3F, 0x41 - 0x46)"
      # "Start of Date Bytes"
      # "Store GIUD command:\n0x29:0x80:0x04:0x80:0x00:0x25:0x64:0x00:0x0B:0xXX:0xXX:0xXX:0xXX:0xXX:0xXX:0xXX:0xXX:0xXX:0xXX:0xXX:0xXX:0xXX:0xXX:0xXX:0xXX:0xXX:0xXX:0xXX:0xXX:0xXX:0xXX:0xXX:0xXX:0xXX:0xXX:0xXX:0xXX:0xXX:0xXX:0xXX:0xXX:"
      n176 = call "Generate GUID.vi"() -> ("GUID"=w518:string)  [unwired: 10 in, 1 out]
      "GUID" <- w518
      n177 = String To Byte Array(string=w518) -> (unsigned byte array=w515:u8[])
      n178 = Insert Into Array(array=u8[] [41, 128, 4, 128, 0, 37, 100, 0, 11], index=9, new element=w515) -> (w514:u8[])
    }
    frame "Cable Auto ID" {
      w521 = TRUE  # Get Response
      w522 = TRUE  # Get ACK/NAK
      # "0x05, 0xA1, 0x04, 0x00, 0x6E"
    }
    frame "Store RSM 627" {
      w524 = FALSE  # Get Response
      w525 = TRUE  # Get ACK/NAK
      # "0x0A, 0xA1, 0x04, 0x80, 0x45, 0x02, 0x73, 0x42, 0x07, 0x02"
    }
    frame "Hall Effect switch" {
      w527 = TRUE  # Get Response
      w528 = TRUE  # Get ACK/NAK
    }
    frame "Read RSM 627" {
      w531 = TRUE  # Get Response
      w530 = TRUE  # Get ACK/NAK
      # "\"0x07, 0xA1, 0x04, 0x80, 0x42,0x02,0x73\""
    }
  }
  n179 = case shown="False" FALSE {
    tunnel: [w533 w537] -> w8
    tunnel: [_ w536] -> w7
    tunnel: "VISA resource name" -> [w533 w534]
    frame False {
    }
    frame True {
      n180 = call "MIMIC Port Init.vi"("MIMIC TIMEOUT"=u32 500, "MIMC BAUD"=u32 9600, "MIMIC_PORT"=w534) -> ("error out"=w536:errorcluster, "MIMIC PORT RESOURCE"=w537:refnum<visa-resource-name>)
    }
  }
  n181 = local write "Array"(w6) -> ()
  n182 = call "XmitMIMICCommand.vi"("error in (no error)"=w7, "HWHSflag"="HWHSflag", "Command array"=w6, "VISA resource name"=w8) -> ("error out"=w22:errorcluster, "VISA resource name Out"=w21:refnum<visa-resource-name>)
  n183 = case shown="False" w27 {
    tunnel: [w541 w545] -> w26
    tunnel: w22 -> [w541 w550]
    tunnel: w21 -> [w540 w548]
    tunnel: [w540 w546] -> w24
    tunnel: [_ w544] -> w16
    tunnel: [w539 w543] -> w15
    tunnel: "wait (ms)" -> [w539 w542]
    frame False {
    }
    frame True {
      # "NEED TO CHECK ACK"
      n184 = flat-sequence {
        tunnel: w550 -> [w553]
        tunnel: [w553] -> w549
        tunnel: w548 -> [w552]
        tunnel: [w552] -> w547
        tunnel: [w551] -> w543
        tunnel: w542 -> [w551]
        tunnel: w549 -> [w558]
        tunnel: w547 -> [w557]
        tunnel: [w556] -> w546
        tunnel: [w555] -> w545
        tunnel: [w554] -> w544
        frame #0 {
          n185 = Wait (ms)(milliseconds to wait=w551) -> ()  [unwired: 1 out]
        }
        frame #1 {
          n186 = call "MIMIC RecvCommand.vi"("error in"=w558, "VISA resource name"=w557) -> ("error out"=w555:errorcluster, "Receive_buffer"=w554:u8[], "VISA resource name OUT"=w556:refnum<visa-resource-name>)  [unwired: 2 in, 1 out]
          n187 = Number To Hexadecimal String(2:w554) -> (0:→"hex integer string":string[])  [unwired: 1 in]
        }
      }
    }
  }
  n188 = case shown="True" w25 {
    tunnel: [w562 w569] -> w17
    tunnel: w26 -> [w562 w564]
    tunnel: w24 -> [w561 w566]
    tunnel: [w560 w570] -> w18
    tunnel: [w561 w568] -> w19
    tunnel: w16 -> [w560 _]
    tunnel: w15 -> [_ w563]
    frame False {
    }
    frame True {
      n189 = flat-sequence {
        tunnel: [w573] -> w567
        tunnel: w566 -> [w573]
        tunnel: [w572] -> w565
        tunnel: w564 -> [w572]
        tunnel: w563 -> [w571]
        tunnel: [w578] -> w570
        tunnel: [w577] -> w569
        tunnel: [w576] -> w568
        tunnel: w567 -> [w574]
        tunnel: w565 -> [w575]
        frame #0 {
          n190 = Wait (ms)(milliseconds to wait=w571) -> ()  [unwired: 1 out]
        }
        frame #1 {
          n191 = call "MIMIC RecvCommand.vi"("error in"=w575, "VISA resource name"=w574) -> ("error out"=w577:errorcluster, "Receive_buffer"=w578:u8[], "VISA resource name OUT"=w576:refnum<visa-resource-name>)  [unwired: 2 in, 1 out]
        }
      }
    }
  }
  n192 = case shown="\"Read FIPSKEY\"" "MIMIC HOST COMMAND" {
    tunnel: w19 -> [w586 w590 w593 w596 w599 w602 w605 w608 w611 w614 w617 w620 w623 w626 w629 w632 w635 w638 w641 w653 w665 w668 w671 w674 w677 w680 w683 w692 w695 w702 w721 w744 w747 w753 w789 w825 w839 w853 w856 w858 w875 w880 w883 w887 w897 w908 w916 w919 w928 w930 w941 w952 w957 w975 w978 w981 w984 w989 w1002]
    tunnel: [w586 w590 w593 w596 w599 w602 w605 w608 w611 w614 w617 w620 w623 w626 w629 w632 w635 w638 w641 w653 w665 w668 w671 w674 w677 w680 w683 w692 w695 w702 w721 w744 w747 w753 w789 w825 w839 w853 w856 w858 w875 w880 w883 w887 w897 w908 w916 w919 w928 w930 w941 w952 w957 w975 w978 w981 w984 w989 w1002] -> w13
    tunnel: w18 -> [w582 w589 w592 w595 w598 w601 w604 w607 w610 w613 w616 w619 w622 w625 w628 w631 w634 w637 w640 w651 w663 w667 w670 w673 w676 w679 w682 w684 w694 w697 w719 w743 w746 w749 w758 w794 w830 w844 w854 w860 w870 w879 w884 w888 w894 w907 w913 w918 w925 w931 w937 w945 w954 w970 w977 w980 w983 w986 w1001]
    tunnel: [w582 w589 w592 w595 w598 w601 w604 w607 w610 w613 w616 w619 w622 w625 w628 w631 w634 w637 w640 w646 w658 w667 w670 w673 w676 w679 w682 w684 w694 w696 w719 w743 w746 w748 w758 w794 w830 w844 w854 w859 w873 w879 w881 w888 w892 w907 w910 w918 w923 w931 w933 w943 w956 w969 w977 w980 w983 w985 w1001] -> w12
    tunnel: w17 -> [w587 w588 w591 w594 w597 w600 w603 w606 w609 w612 w615 w618 w621 w624 w627 w630 w633 w636 w639 w652 w664 w666 w669 w672 w675 w678 w681 w691 w693 w701 w722 w742 w745 w752 w788 w824 w838 w852 w855 w857 w874 w878 w882 w889 w898 w906 w917 w920 w929 w932 w940 w953 w958 w974 w976 w979 w982 w988 w1000]
    tunnel: [w587 w588 w591 w594 w597 w600 w603 w606 w609 w612 w615 w618 w621 w624 w627 w630 w633 w636 w639 w652 w664 w666 w669 w672 w675 w678 w681 w691 w693 w701 w722 w742 w745 w752 w788 w824 w838 w852 w855 w857 w874 w878 w882 w889 w898 w906 w917 w920 w929 w932 w940 w953 w958 w974 w976 w979 w982 w988 w1000] -> w11
    tunnel: [w584 _ _ _ _ _ _ _ _ _ _ _ _ _ _ _ _ _ _ w647 w659 _ _ _ _ _ _ w688 _ _ w724 _ _ _ w759 w795 w826 w840 _ _ w871 _ _ _ w890 w900 w911 _ w921 _ w935 w944 _ w967 _ _ _ _ _] -> w9
    frame "Enter FAT", Default {
      n193 = Array Subset(array=w582, index=5, length=200) -> (w581:u8[])
      n194 = Byte Array To String(unsigned byte array=w581) -> (string=w585:string)
      n195 = local read "Receive_Unpacked_Data"() -> (w583:T1)
      n196 = Bundle By Name(cluster=w583, "Response_String_1"=w585) -> (w584:T1)
    }
    frame "Beeper Control" {
    }
    frame "ParamSend" {
    }
    frame "General" {
    }
    frame "General-Response" {
    }
    frame "RSM Init" {
    }
    frame "RSM EnterFAT" {
    }
    frame "RSM - SE4500 - Peek PRISM Register GENERIC command" {
    }
    frame "RSM - SE4500 - Poke PRISM Register GENERIC command" {
    }
    frame "RSM - SE4500 - GENERIC command" {
    }
    frame "RSM - SE4500 - SetPDM Calibration" {
    }
    frame "RSM - SE4500 - SetPDM-Z Calibration" {
    }
    frame "LED On" {
    }
    frame "Image Mode" {
    }
    frame "Start Session" {
    }
    frame "Stop Session" {
    }
    frame "Change Buadrate" {
    }
    frame "Auto Exposure" {
    }
    frame "Set Manual Exposure" {
    }
    frame "Read BT Address" {
      n197 = Array Subset(array=w651, index=14, length=6) -> (w646:u8[])
      n198 = Number To Hexadecimal String(1:i16 2 ("width (-)"), 2:w646) -> (0:w644:string[])
      n199 = local read "Receive_Unpacked_Data"() -> (w648:T1)
      n200 = Concatenate Strings(w644, "" ("string")) -> (w643:string)
      n201 = Bundle By Name(cluster=w648, "Response_String_1"=w643) -> (w647:T1)
    }
    frame "Read FIPSKEY" {
      n202 = Array Subset(array=w663, index=14, length=16) -> (w658:u8[])
      n203 = Number To Hexadecimal String(1:i16 2 ("width (-)"), 2:w658) -> (0:w656:string[])
      n204 = local read "Receive_Unpacked_Data"() -> (w660:T1)
      n205 = Concatenate Strings(w656, "" ("string")) -> (w655:string)
      n206 = Bundle By Name(cluster=w660, "Response_String_1"=w655) -> (w659:T1)
    }
    frame "Store BT Address" {
    }
    frame "Store FIPSKEY" {
    }
    frame "Pairing Command" {
    }
    frame "Un-Pairing" {
    }
    frame "Set Illumination" {
    }
    frame "Set Defaults" {
    }
    frame "Exit FAT" {
      n207 = Array Subset(array=w684, index=5, length=13) -> (w685:u8[])
      n208 = Byte Array To String(unsigned byte array=w685) -> (string=w690:string)
      n209 = local read "Receive_Unpacked_Data"() -> (w689:T1)
      n210 = Bundle By Name(cluster=w689, "Response_String_1"=w690) -> (w688:T1)
    }
    frame "LED Off" {
    }
    frame "Trigger" {
      n211 = Empty Array?(array=w697) -> (empty?=w698:bool)
      n212 = case shown="False" w698 {
        tunnel: w697 -> [w704 _]
        tunnel: [w703 w710] -> w696
        frame False {
          n213 = Array Subset(array=w704, index=5, length=1) -> (w703:u8[])
        }
        frame True {
          # "If empty, init array and set its values to zero."
          n214 = To Unsigned Byte Integer(number=u8 0) -> (unsigned 8bit integer=w708:u8)
          n215 = Initialize Array(w708, 1 ("dimension size")) -> (w710:u8[])
        }
      }
      n216 = Array Subset(array=w697, index=5, length=1) -> ()  [unwired: 1 out]
    }
    frame "Imager Time To Decode Test" {
      n217 = Byte Array To String(unsigned byte array=w719) -> (string=w735:string)
      n218 = Replace Substring(2:17 ("length (len. of substring)"), 3:0 ("offset (0)"), 5:w735) -> (1:w730:string)  [unwired: 1 in, 1 out]
      n219 = String Length(string=w730) -> (length=w729:i32)
      n220 = Index Array(array=w719, index=5) -> (element=w732:u8)
      n221 = Subtract(x=w729, y=2) -> (x-y=w727:i32)
      n222 = Index Array(array=w719, index=7 ("length")) -> (element=w714:u8)
      n223 = Index Array(array=w719, index=6) -> (element=w717:u8)
      n224 = case shown="1" w732 {
        frame 0, Default {
          n225 = local read "Receive_Unpacked_Data"() -> (w736:T1)
          n226 = Bundle By Name(cluster=w736, "Decode_Status"="No Decode" ("Decode_Data")) -> (w737:T1)
          n227 = local write "Receive_Unpacked_Data"(w737) -> ()
        }
        frame 1 {
          n228 = local read "Receive_Unpacked_Data"() -> (w740:T1)
          n229 = Bundle By Name(cluster=w740, "Decode_Status"="SUCCESS" ("Decode_Data")) -> (w739:T1)
          n230 = local write "Receive_Unpacked_Data"(w739) -> ()
        }
      }
      n231 = Join Numbers(hi=u8 0, lo=w717) -> ((hi.lo)=w712:u16)
      n232 = Join Numbers(hi=w714, lo=u8 0 ("hi")) -> ((hi.lo)=w713:u16)
      n233 = Add(x=w712, y=w713) -> (x+y=w711:u16)
      n234 = local write "TimeToDecode"(w711) -> ()
      n235 = Replace Substring(2:2 ("length (len. of substring)"), 3:w727, 5:w730) -> (1:w725:string)  [unwired: 1 in, 1 out]
      n236 = local read "Receive_Unpacked_Data"() -> (w723:T1)
      n237 = Bundle By Name(cluster=w723, "Decode_Data"=w725, "Time_To_Decode"=w711) -> (w724:T1)
    }
    frame "Battery Off" {
    }
    frame "Battery Charge Control" {
    }
    frame "Read Battery Voltage" {
      # "Voltage (MSB_LSB *.0006*2)"
      # "RESPONSE\nLength Byte:\t0x0D\nOpcode Byte:\t0x21\nSource Byte:\t0x00\nStatus Byte:\t0x80\nSub-opcode Byte:\t0x42\nData Byte 1:\t0x75: Attribute MSB\nData Byte 2:\t0x30: Attribute LSB\nData Byte 3:\t0x57: Attribute is Word ('W') value\nData Byte 4:\t0x01\nData Byte 5:\t0xXX: Battery Voltage MSB\nData Byte 6:\t0xXX: Battery Voltage LSB\nData Byte 7:\t0xFF: Packet Termination\nData Byte 8:\t0xFF: Packet Termination\nChecksum High Byte:\t0xXX\nChecksum Low Byte:\t0xXX"
      n238 = Array Subset(array=w749, index=0, length=15) -> (w748:u8[])
    }
    frame "RSM - SE4500 - GetPDM Calibration" {
      n239 = Index Array(array=w758, index=14) -> (element=w784:u8)
      n240 = Index Array(array=w758, index=16) -> (element=w777:u8)
      n241 = Index Array(array=w758, index=13) -> (element=w785:u8)
      n242 = Index Array(array=w758, index=15) -> (element=w778:u8)
      n243 = Index Array(array=w758, index=18) -> (element=w770:u8)
      n244 = Index Array(array=w758, index=20) -> (element=w764:u8)
      n245 = Index Array(array=w758, index=17) -> (element=w771:u8)
      n246 = Index Array(array=w758, index=19) -> (element=w765:u8)
      n247 = Join Numbers(hi=w784, lo=w785) -> ((hi.lo)=w757:u16)
      n248 = Join Numbers(hi=w777, lo=w778) -> ((hi.lo)=w754:u16)
      n249 = Join Numbers(hi=w770, lo=w771) -> ((hi.lo)=w755:u16)
      n250 = Join Numbers(hi=w764, lo=w765) -> ((hi.lo)=w756:u16)
      n251 = Number To Decimal String(number=w757, width (-)=i16 4) -> (decimal integer string=w783:string)
      n252 = Number To Decimal String(number=w754, width (-)=i16 4) -> (decimal integer string=w776:string)
      n253 = Number To Decimal String(number=w755, width (-)=i16 4) -> (decimal integer string=w769:string)
      n254 = Number To Decimal String(number=w756, width (-)=i16 4) -> (decimal integer string=w763:string)
      n255 = local read "Receive_Unpacked_Data"() -> (w781:T1)
      n256 = Bundle By Name(cluster=w781, "Response_String_1"=w783) -> (w774:T1)
      n257 = Bundle By Name(cluster=w774, "Response_String_2"=w776) -> (w761:T1)
      n258 = Bundle By Name(cluster=w761, "Response_String_3"=w769) -> (w760:T1)
      n259 = Bundle By Name(cluster=w760, "Response_String_4"=w763) -> (w759:T1)
    }
    frame "RSM - SE4500 - GetPDM-Z Calibration" {
      n260 = Index Array(array=w794, index=14) -> (element=w820:u8)
      n261 = Index Array(array=w794, index=16) -> (element=w813:u8)
      n262 = Index Array(array=w794, index=13) -> (element=w821:u8)
      n263 = Index Array(array=w794, index=15) -> (element=w814:u8)
      n264 = Index Array(array=w794, index=22) -> (element=w806:u8)
      n265 = Index Array(array=w794, index=24) -> (element=w800:u8)
      n266 = Index Array(array=w794, index=21) -> (element=w807:u8)
      n267 = Index Array(array=w794, index=23) -> (element=w801:u8)
      n268 = Join Numbers(hi=w820, lo=w821) -> ((hi.lo)=w793:u16)
      n269 = Join Numbers(hi=w813, lo=w814) -> ((hi.lo)=w790:u16)
      n270 = Join Numbers(hi=w806, lo=w807) -> ((hi.lo)=w791:u16)
      n271 = Join Numbers(hi=w800, lo=w801) -> ((hi.lo)=w792:u16)
      n272 = Number To Decimal String(number=w793, width (-)=i16 4) -> (decimal integer string=w819:string)
      n273 = Number To Decimal String(number=w790, width (-)=i16 4) -> (decimal integer string=w812:string)
      n274 = Number To Decimal String(number=w791, width (-)=i16 4) -> (decimal integer string=w805:string)
      n275 = Number To Decimal String(number=w792, width (-)=i16 4) -> (decimal integer string=w799:string)
      n276 = local read "Receive_Unpacked_Data"() -> (w817:T1)
      n277 = Bundle By Name(cluster=w817, "Response_String_1"=w819) -> (w810:T1)
      n278 = Bundle By Name(cluster=w810, "Response_String_2"=w812) -> (w797:T1)
      n279 = Bundle By Name(cluster=w797, "Response_String_3"=w805) -> (w796:T1)
      n280 = Bundle By Name(cluster=w796, "Response_String_4"=w799) -> (w795:T1)
    }
    frame "Get Object Sensor Value" {
      n281 = Index Array(array=w830, index=5) -> (element=w829:u8)
      n282 = Index Array(array=w830, index=6) -> (element=w828:u8)
      n283 = Number To Hexadecimal String(1:i16 2 ("width (-)"), 2:w829) -> (0:w837:string)
      n284 = Number To Hexadecimal String(1:i16 2 ("width (-)"), 2:w828) -> (0:w833:string)
      n285 = local read "Receive_Unpacked_Data"() -> (w835:T1)
      n286 = Bundle By Name(cluster=w835, "Response_String_1"=w837) -> (w831:T1)
      n287 = Bundle By Name(cluster=w831, "Response_String_2"=w833) -> (w826:T1)
    }
    frame "Read Object Sensor Calibration Value" {
      n288 = Index Array(array=w844, index=9) -> (element=w843:u8)
      n289 = Index Array(array=w844, index=10) -> (element=w842:u8)
      n290 = Number To Hexadecimal String(1:i16 2 ("width (-)"), 2:w843) -> (0:w851:string)
      n291 = Number To Hexadecimal String(1:i16 2 ("width (-)"), 2:w842) -> (0:w847:string)
      n292 = local read "Receive_Unpacked_Data"() -> (w849:T1)
      n293 = Bundle By Name(cluster=w849, "Response_String_1"=w851) -> (w845:T1)
      n294 = Bundle By Name(cluster=w845, "Response_String_2"=w847) -> (w840:T1)
    }
    frame "Store Object Sensor Calibration Value" {
    }
    frame "Read Battery Temperature" {
      # "RESPONSE\nLength Byte:\t0x0D\nOpcode Byte:\t0x21\nSource Byte:\t0x00\nStatus Byte:\t0x80\nSub-opcode Byte:\t0x42\nData Byte 1:\t0x75: Attribute MSB\nData Byte 2:\t0x31: Attribute LSB\nData Byte 3:\t0x57: Attribute is Word ('W') value\nData Byte 4:\t0x01\nData Byte 5:\t0xXX: Battery Temperature MSB\nData Byte 6:\t0xXX: Battery Temperature LSB\nData Byte 7:\t0xFF: Packet Termination\nData Byte 8:\t0xFF: Packet Termination\nChecksum High Byte:\t0xXX\nChecksum Low Byte:\t0xXX"
      n295 = Array Subset(array=w860, index=0, length=15) -> (w859:u8[])
    }
    frame "Software Version" {
      n296 = Array Subset(array=w870, index=32, length=16) -> (w867:u8[])
      n297 = Array Subset(array=w870, index=13, length=16) -> (w873:u8[])
      n298 = Byte Array To String(unsigned byte array=w873) -> (string=w866:string)
      n299 = Byte Array To String(unsigned byte array=w867) -> (string=w865:string)
      n300 = Concatenate Strings(w866, "  " ("string"), w865) -> (w863:string)
      n301 = local read "Receive_Unpacked_Data"() -> (w872:T1)
      n302 = Bundle By Name(cluster=w872, "Code_Revision"=w863) -> (w871:T1)
    }
    frame "StoreFeatureSet" {
    }
    frame "ReadFeatureSet" {
      # "Feature Set Responce:\n0x0C, 0x21, 0x00, 0x00, 0x42, 0x02, 0xC2,0x42,0x01,\n\t\t\t\t\t\t\t\t\t\t\t  \t\t\t  0xff, //FEATURE-SET\n\t\t\t\t\t\t\t\t\t\t\t\t\t\t  0xff,0xff, // packet termination\n\t\t\t\t\t\t\t\t\t\t\t\t\t\t  0x00, 0x00}; //checksum"
      n303 = Array Subset(array=w884, index=9, length=1) -> (w881:u8[])
    }
    frame "Store Model Number" {
    }
    frame "Read Model Number" {
      n304 = Array Subset(array=w894, index=13, length=18) -> (w892:u8[])
      n305 = Byte Array To String(unsigned byte array=w892) -> (string=w893:string)
      n306 = local read "Receive_Unpacked_Data"() -> (w891:T1)
      n307 = Bundle By Name(cluster=w891, "Response_String_1"=w893) -> (w890:T1)
    }
    frame "Store Manufacturing Date" {
      n308 = Get Date/Time In Seconds() -> (seconds since 1Jan1904=w905:timestamp)
      n309 = Format Date/Time String(time format string (%c)="%d%b%y", seconds (now)=w905, UTC format=FALSE) -> (date/time string=w902:string)
      n310 = To Upper Case(1:w902) -> (0:w899:string)
      n311 = local read "Receive_Unpacked_Data"() -> (w901:T1)
      n312 = Bundle By Name(cluster=w901, "Response_String_1"=w899) -> (w900:T1)
    }
    frame "Read Manufacturing Date" {
      n313 = Array Subset(array=w913, index=13, length=7) -> (w910:u8[])
      n314 = Byte Array To String(unsigned byte array=w910) -> (string=w912:string)
      n315 = local read "Receive_Unpacked_Data"() -> (w909:T1)
      n316 = Bundle By Name(cluster=w909, "Response_String_1"=w912) -> (w911:T1)
    }
    frame "Store Service Date" {
    }
    frame "Read Service Date" {
      n317 = Array Subset(array=w925, index=13, length=7) -> (w923:u8[])
      n318 = Byte Array To String(unsigned byte array=w923) -> (string=w924:string)
      n319 = local read "Receive_Unpacked_Data"() -> (w922:T1)
      n320 = Bundle By Name(cluster=w922, "Response_String_1"=w924) -> (w921:T1)
    }
    frame "Store Serial Number" {
    }
    frame "Read Serial Number" {
      n321 = Array Subset(array=w937, index=13, length=16) -> (w933:u8[])
      n322 = Byte Array To String(unsigned byte array=w933) -> (string=w936:string)
      n323 = local read "Receive_Unpacked_Data"() -> (w934:T1)
      n324 = Bundle By Name(cluster=w934, "Response_String_1"=w936) -> (w935:T1)
    }
    frame "Query Paired Address" {
      # "Cradle BT Address"
      # "Pair Status\n0x00: Unpaired \n0x01: Paired"
      n325 = Array Subset(array=w945, index=6, length=6) -> (w948:u8[])
      n326 = Array Subset(array=w945, index=5, length=1) -> (w943:u8[])
      n327 = local read "Receive_Unpacked_Data"() -> (w942:T1)
      n328 = Byte Array To String(unsigned byte array=w948) -> (string=w949:string)
      n329 = Bundle By Name(cluster=w942, "Response_String_1"=w949) -> (w944:T1)
    }
    frame "Pairing Status" {
      # "Pairing Status\n0x00: Cradle is not paired\n0x01: Cradle is paired"
      n330 = Empty Array?(array=w954) -> (empty?=w955:bool)
      n331 = case shown="False" w955 {
        tunnel: w954 -> [w960 _]
        tunnel: [w959 w966] -> w956
        frame False {
          n332 = Array Subset(array=w960, index=5, length=1) -> (w959:u8[])
        }
        frame True {
          # "If empty, init array and set its values to zero."
          n333 = To Unsigned Byte Integer(number=u8 0) -> (unsigned 8bit integer=w964:u8)
          n334 = Initialize Array(w964, 1 ("dimension size")) -> (w966:u8[])
        }
      }
    }
    frame "Read GUID" {
      n335 = Array Subset(array=w970, index=5, length=32) -> (w969:u8[])
      n336 = Byte Array To String(unsigned byte array=w969) -> (string=w973:string)
      n337 = local read "Receive_Unpacked_Data"() -> (w968:T1)
      n338 = Bundle By Name(cluster=w968, "Response_String_1"=w973) -> (w967:T1)
    }
    frame "Cable Auto ID" {
    }
    frame "Store RSM 627" {
    }
    frame "Store GUID " {
    }
    frame "Hall Effect switch" {
      n339 = Empty Array?(array=w986) -> (empty?=w987:bool)
      n340 = case shown="True" w987 {
        tunnel: w986 -> [w993 _]
        tunnel: [w992 w999] -> w985
        frame False {
          n341 = Array Subset(array=w993, index=5, length=1) -> (w992:u8[])
        }
        frame True {
          # "If empty, init array and set its values to zero."
          n342 = To Unsigned Byte Integer(number=u8 0) -> (unsigned 8bit integer=w997:u8)
          n343 = Initialize Array(w997, 1 ("dimension size")) -> (w999:u8[])
        }
      }
      n344 = Array Subset(array=w986, index=5, length=1) -> ()  [unwired: 1 out]
    }
    frame "Read RSM 627" {
    }
  }
  "error out" <- w11
  "Receive_buffer" <- w12
  "VISA resource name OUT" <- w13
  "Receive_Unpacked_Data" <- w9
  "TimeToDecode" <- u16 0 ("TimeToDecode")
